vi "Main.vi"() -> ()   [LabVIEW 2013]
doc: "This template is for the Queued Message Handler design pattern.\n\nThe Event Handling Loop generates messages based on user interface actions.\n\nThe Message Handling Loop processes messages generated by the Event Handling Loop, or by other messages. The messages are string values, so new messages can be added easily to the Message Cases case structure in the Message Handling Loop. Each message cluster can also provide an optional value for Message Data, which is a variant that can be converted to whatever message-specific data is required."
uses:
  <vilib>/vision/Image Controls.llb/IMAQ Image.ctl
  Message Passing/MsgQ Loops enum.ctl
  Image Processing/Mask ROI FG Enum.ctl
  System Status/Status FG Enum.ctl
  Globals/Average Sector Data.vi
  controls/UI Data.ctl
  Message Queue/Message Queue.lvlib
  User Event - Stop/User Event - Stop.lvlib
  FPGA/FPGA Frame Grabbing.lvlib
  Image Processing/Image Processing.lvlib
  Common/State Machines/State Machine Lib.lvlib
  Message Passing/Main MsgQ.lvlib
  Common/GUI/GUI.lvlib
  <vilib>/rvi/interface/nirviReadWriteControl/nirviReadWriteControl.xnode
  FGs/FPGA_Reference.ctl
  FPGA Bitfiles/Simulation_WBA.lvbitx
  <vilib>/rvi/errors/niLvFpgaMergeErrorWithErrorCode.vi
  NiFpgaLv.dll
  <vilib>/rvi/errors/niLvFpgaAdjustHostInterfaceError.vi
panel:
  out "Analysis Ticks":u32
  out "Accumulate Ticks":u32
  out "FPGA Display Image":T1(plugin-control)
  out "Right Wingbeat Avg Graph":u8[](graph)
  in  "Start Serial Server":bool=TRUE
  out "Left Wingbeat Avg Graph":u8[](graph)
  in  "Stop Charts":bool
  in  "Wing ROIs":T2
  out "FPGA image info":T5={"Image Type"=0, "Unit"=enum."Undefined", "X Resolution"=2040, "Y Resolution"=1088, "X Step"=1.0, "Y Step"=1.0, "Image Name"="Image"} {"Image Type" items=["Grayscale (U8)", "Grayscale (I16)", "Grayscale (SGL)", "Complex (CSG)", "RGB (U32)", "HSL (U32)", "RGB (U64)", "Grayscale (U16)"]}
  in  "Stream?":bool
  out "FPGA Image":T1
  in  "Test Visual Response":bool
  in  "Test FPGA":bool
  out "Status Update":string="VI Stopped"
  in  "Define Mask":bool
  in  "Acquire Image":bool
  in  "Stop":bool
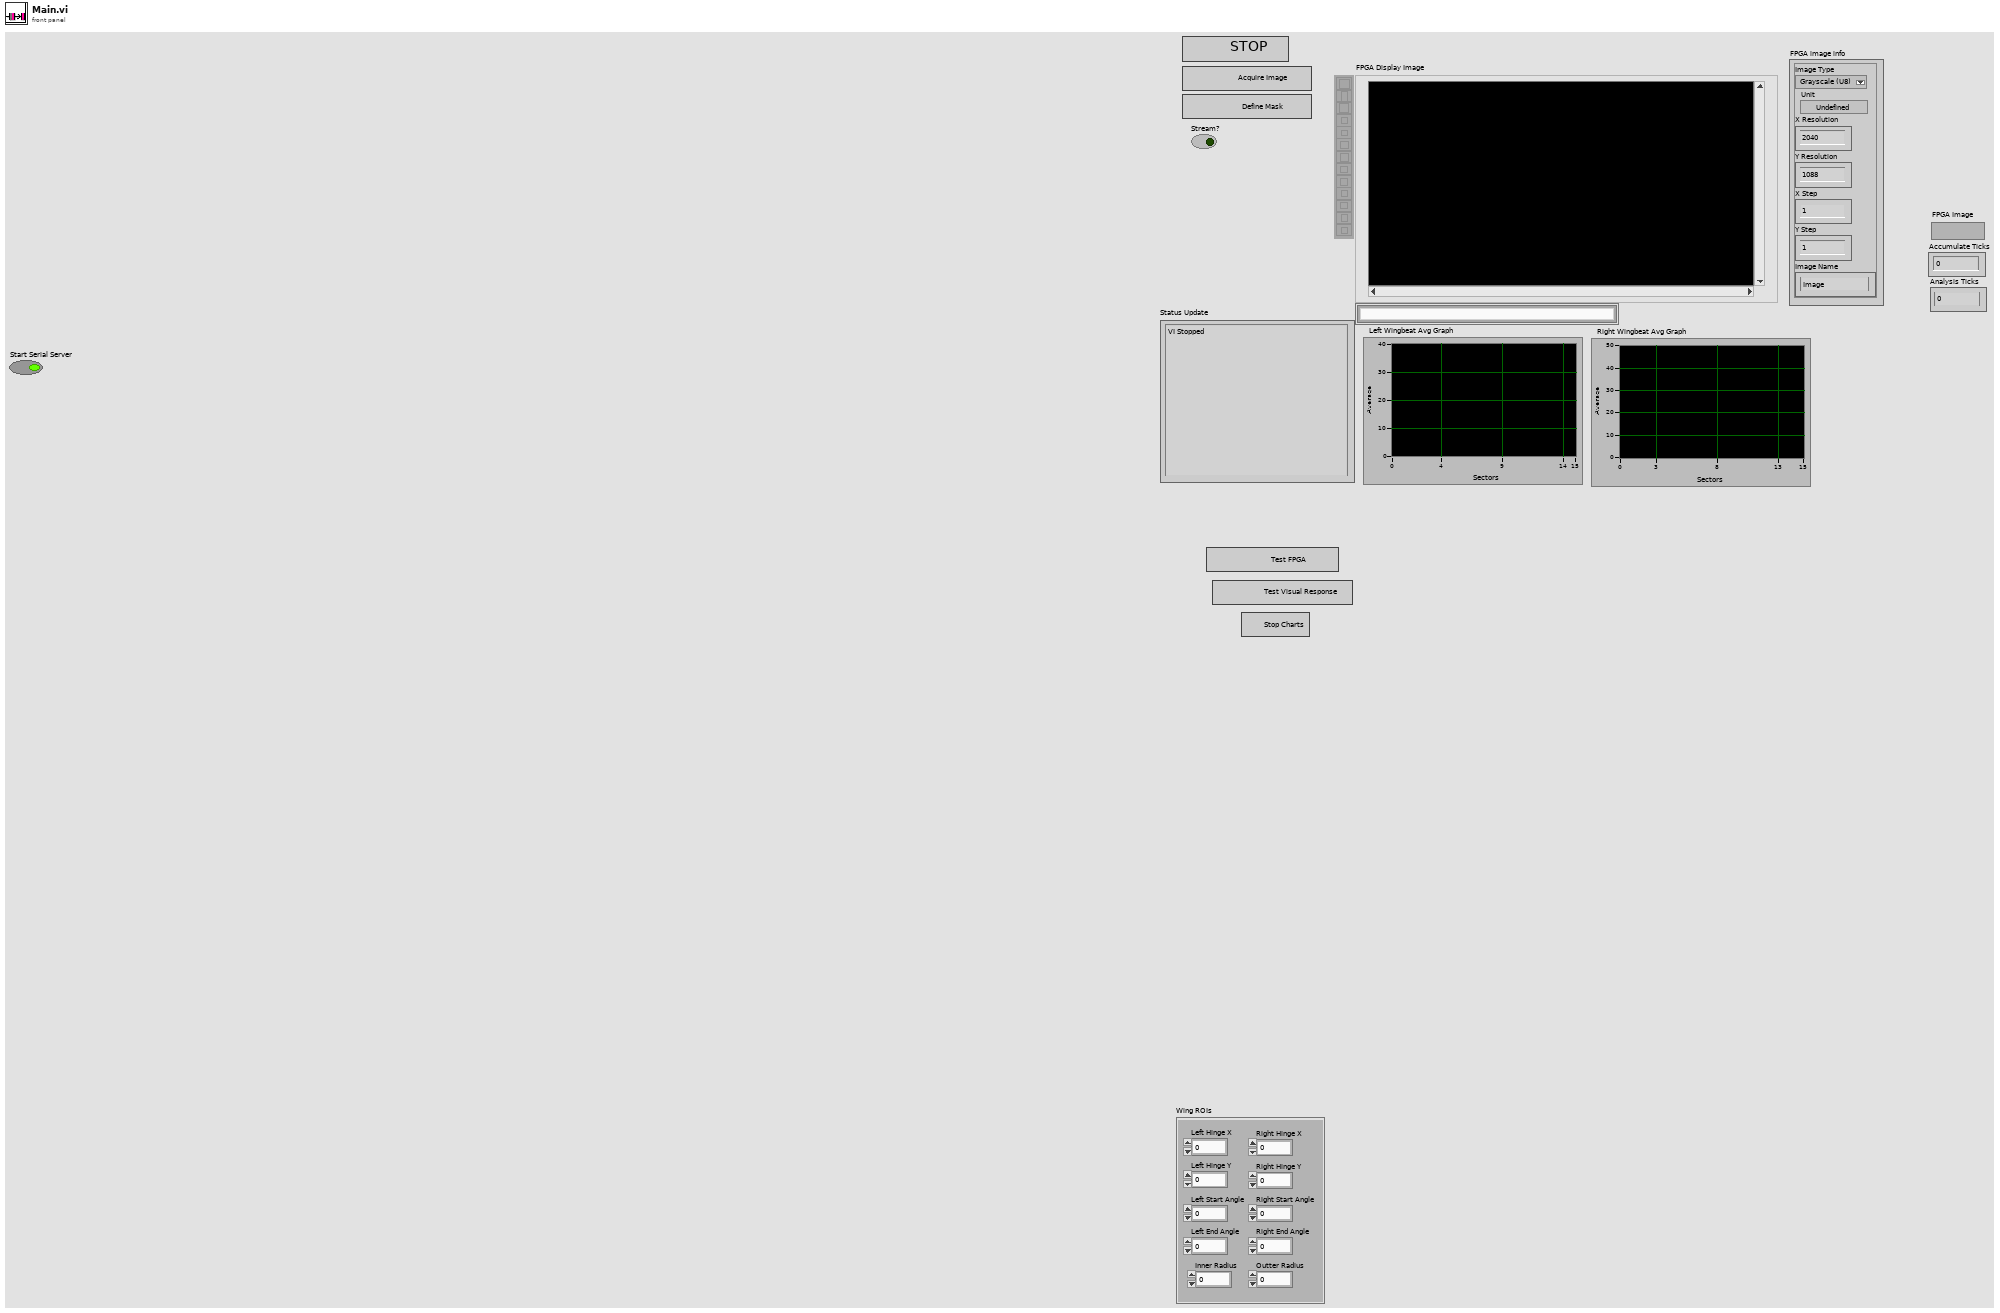
[diagram p1: front panel]
types:
  T1 = typedef "IMAQ Image.ctl" = refnum<image>
  T2 = cluster{"Left Hinge X":u16, "Left Hinge Y":u16, "Inner Radius":u16, "Outter Radius":u16, "Right Hinge X":u16, "Right Hinge Y":u16, "Right Start Angle":i16, "Right End Angle":i16, "Left Start Angle":i16, "Left End Angle":i16}
  T3 = typedef "Image Type" = u32
  T4 = typedef "Image Unit" = enum32{"Undefined", "Angström", "Micrometer", "Millimeter", "Centimeter", "Meter", "Kilometer", "Microinch", "Inch", "Feet", "Nautical miles", "Standard miles", "Steps"}
  T5 = cluster{"Image Type":T3, "Unit":T4, "X Resolution":i32, "Y Resolution":i32, "X Step":sgl, "Y Step":sgl, "Image Name":string}
  T6 = typedef "State Machine Lib.lvlib/STATE cluster.ctl" = cluster{"State":string, "Parameters":variant}
  T7 = typedef "Main MsgQ.lvlib/MsgQ Loops enum.ctl" = enum16{"User Interface", "Image Acq"}
  T8 = typedef "Status FG Enum.ctl" = enum16{"Reset", "Read", "Write"}
  T9 = typedef "Mask ROI FG Enum.ctl" = enum16{"Read", "Write"}
  T10 = typedef "FPGA_Reference.ctl" = refnum<k20>
  T11 = typedef "Mask ROI Cluster.ctl" = cluster{"left annulus":T12, "right annulus":T12, "Threshold Range":cluster{"Lower value":dbl, "Upper value":dbl}, "[Avg BG]":u8[], "Number of Sectors":u8, "Left ROI":T13, "Right ROI":T13, "Left Start Angle Duty Cycle":fxp<+,8,0>, "Left End Angle Duty Cycle":fxp<+,8,0>, "Right End Angle Duty Cycle":fxp<+,8,0>, "Right Start Angle Duty Cycle":fxp<+,8,0>, "[Sector ROIs]":T13[]}
  T12 = typedef "IMAQ Circle" = cluster{"Center X":i32, "Center Y":i32, "Inner Radius":i32, "Outer Radius":i32, "Start Angle":dbl, "End Angle":dbl}
  T13 = typedef "ROI Descriptor" = cluster{"Global Rectangle":i32[], "Contours":cluster{"ID":enum32{"External", "Internal"}, "Type":u32, "Coordinates":i32[]}[]}
  T14 = typedef "UI Data.ctl" = cluster{"Boolean <Replace Me>":bool, "Initial Message":string, "Numeric <Replace Me>":dbl, "Acquire Image Ref":refnum<vi>, "Define Mask Ref":refnum<vi>, "Status Update Ref":refnum<vi>, "Stop Button Ref":refnum<vi>, "FPGA Image":T1, "Processed Image":T1, "Left Annulus":cluster{"Center X":i32, "Center Y":i32, "Inner Radius":i32, "Outer Radius":i32, "Start Angle":dbl, "End Angle":dbl}, "Right Annulus":cluster{"Center X":i32, "Center Y":i32, "Inner Radius":i32, "Outer Radius":i32, "Start Angle":dbl, "End Angle":dbl}}
  T15 = typedef "Message Queue.lvlib/All Message Queues.ctl" = cluster{"UI":refnum<queue>}
  T16 = cluster{"Center X":i32, "Center Y":i32, "Inner Radius":i32, "Outer Radius":i32, "Start Angle":dbl, "End Angle":dbl}
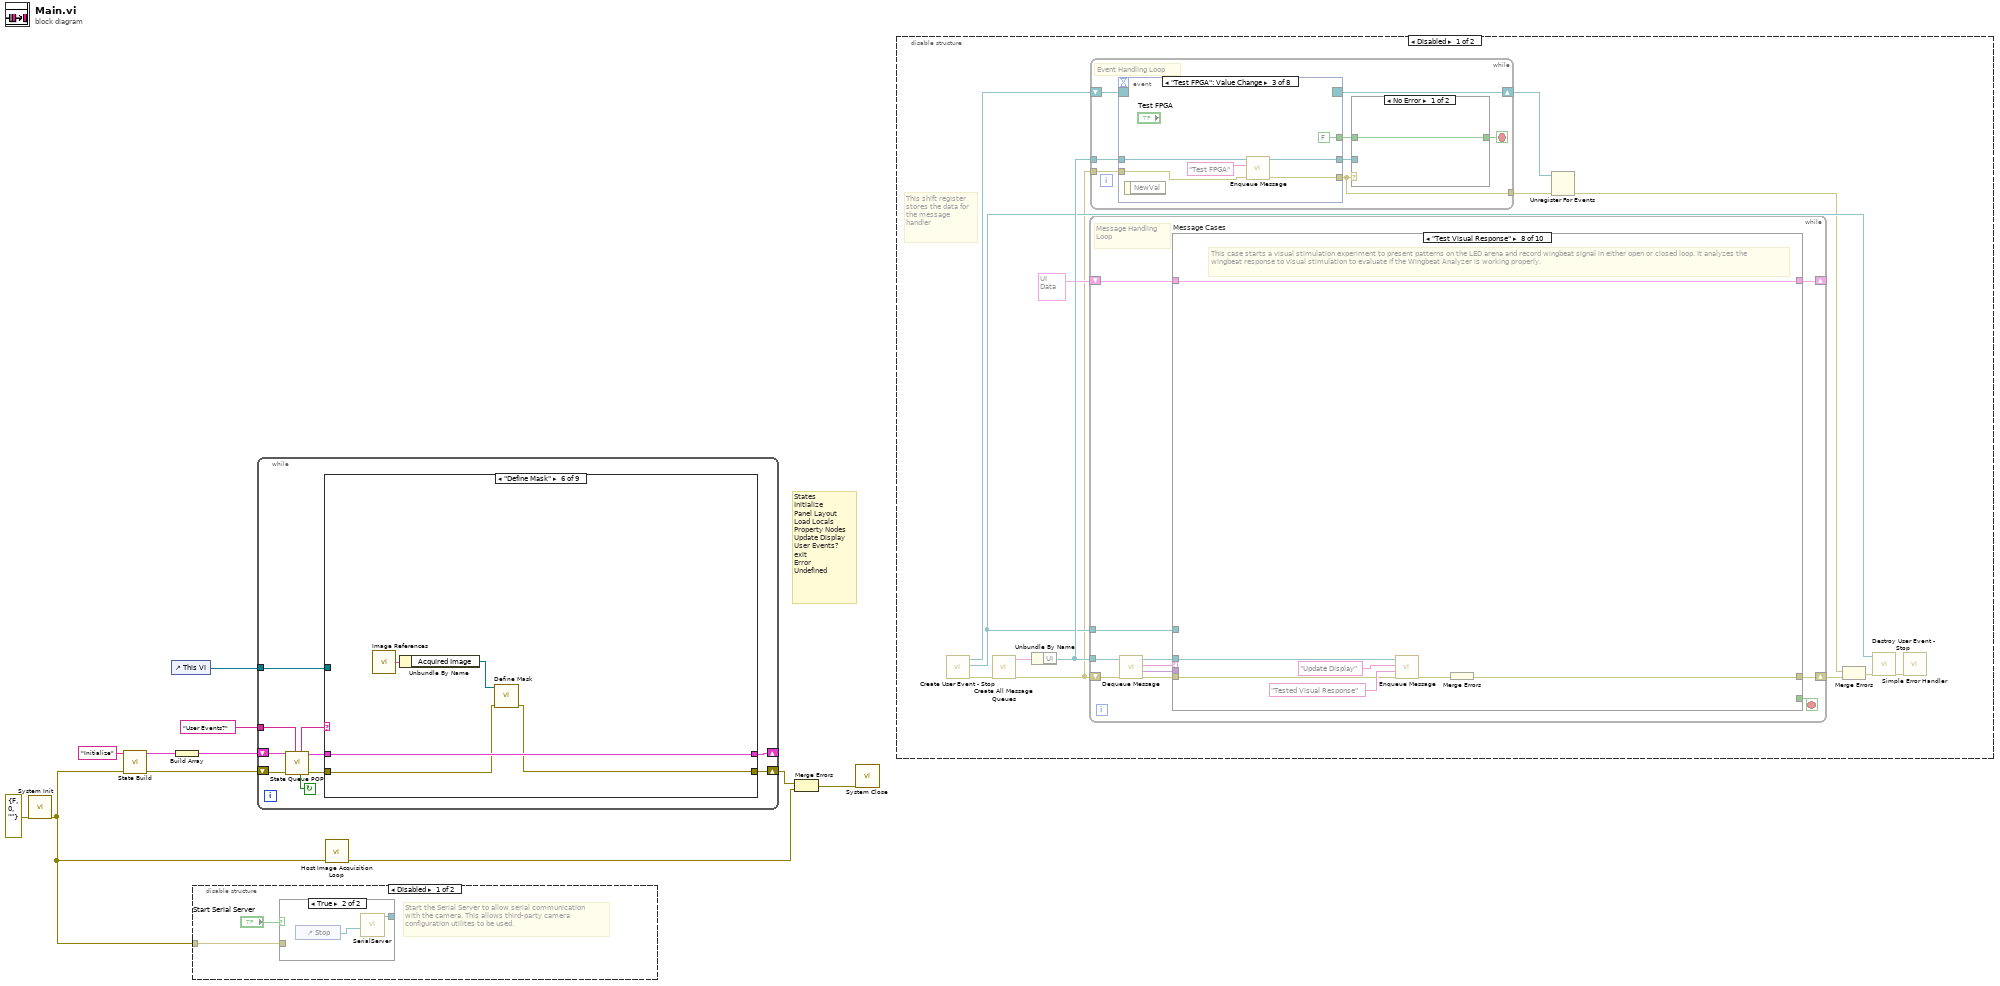
[diagram p0: block diagram]
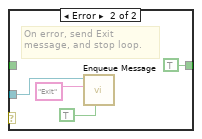
[diagram p4: hidden frame]
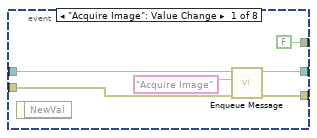
[diagram p5: hidden frame]
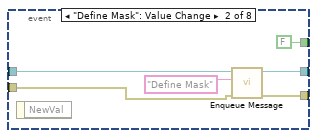
[diagram p6: hidden frame]
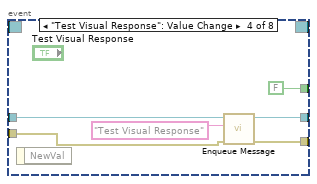
[diagram p7: hidden frame]
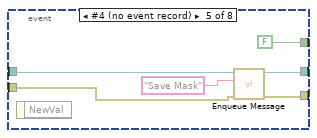
[diagram p8: hidden frame]
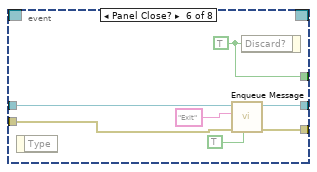
[diagram p9: hidden frame]
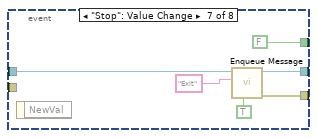
[diagram p10: hidden frame]
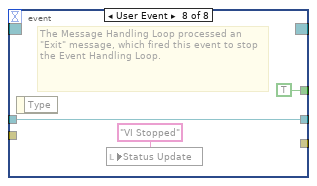
[diagram p11: hidden frame]
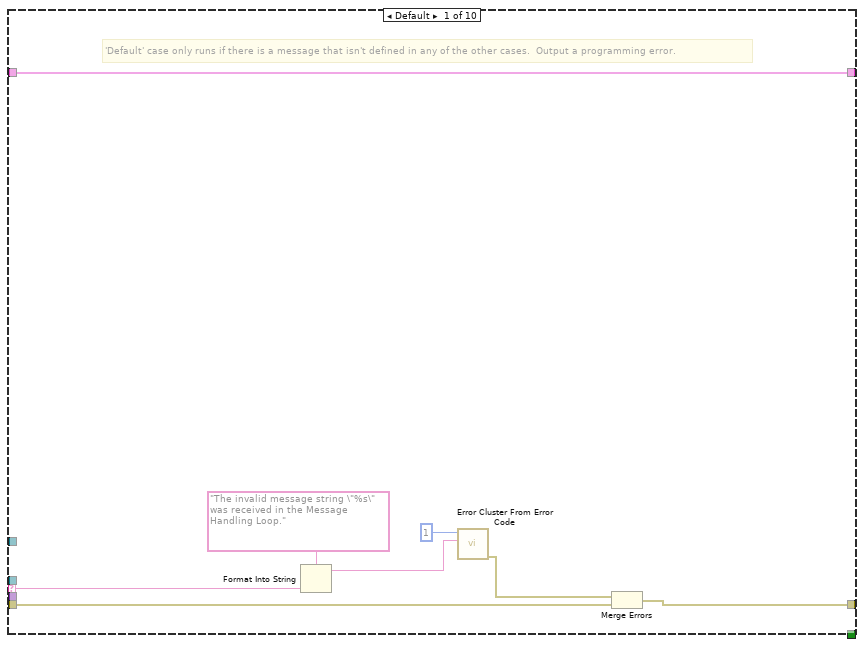
[diagram p12: hidden frame]
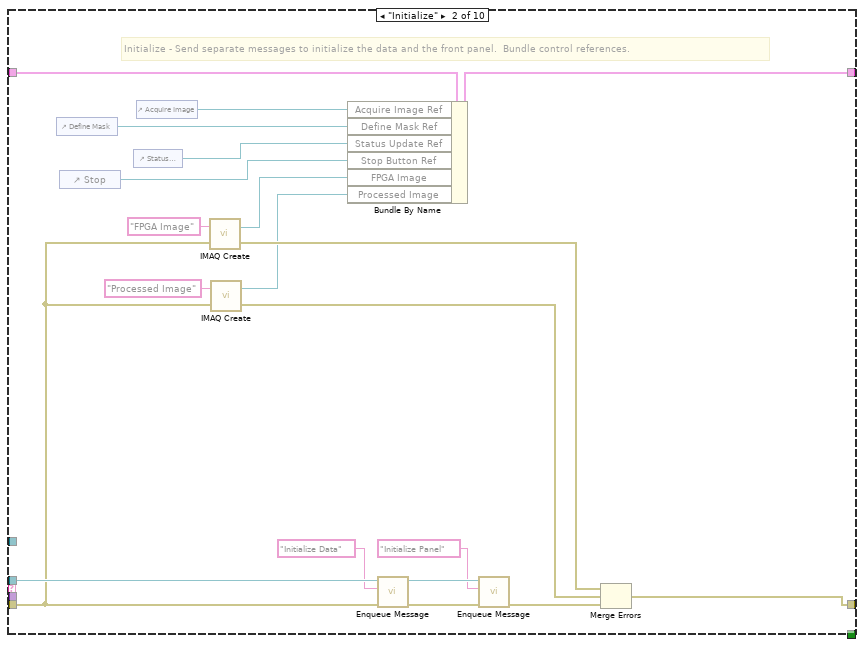
[diagram p13: hidden frame]
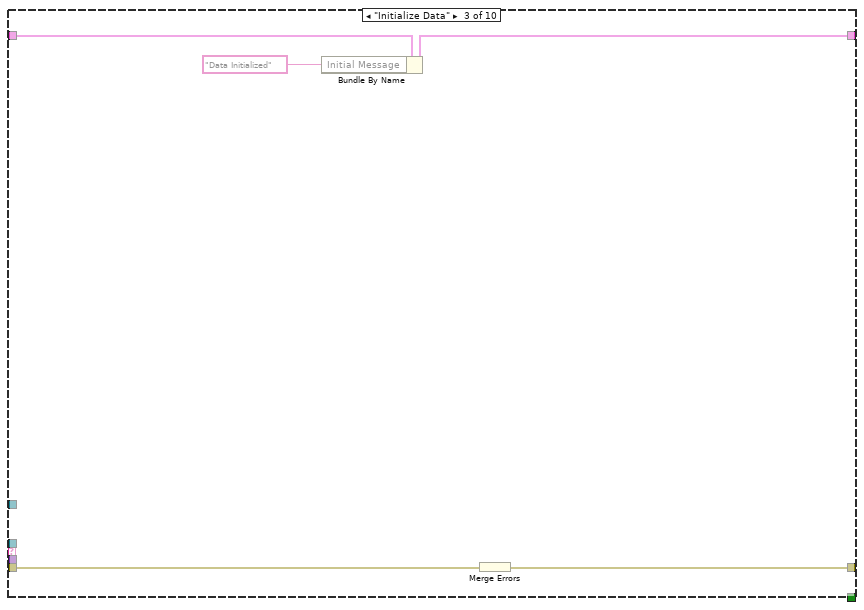
[diagram p14: hidden frame]
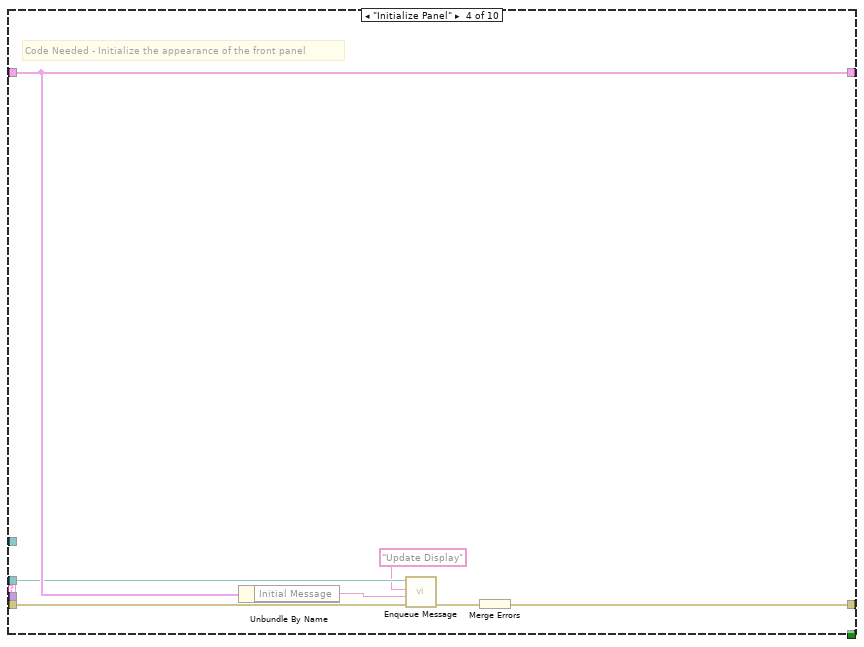
[diagram p15: hidden frame]
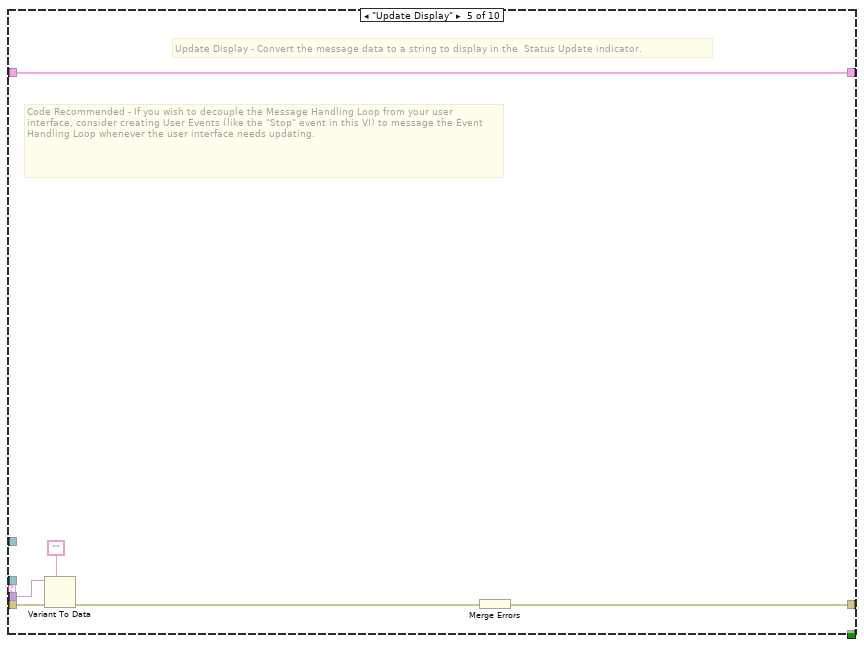
[diagram p16: hidden frame]
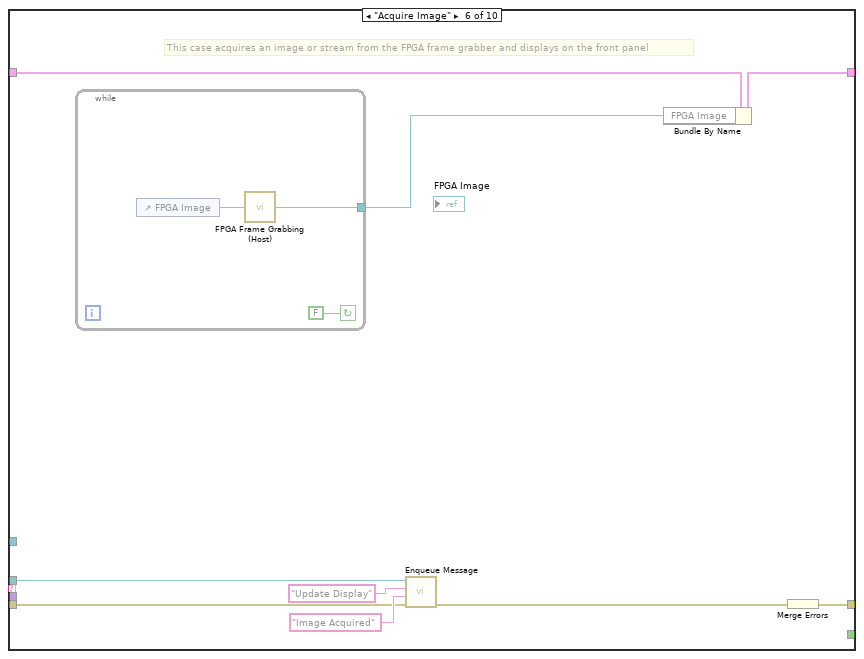
[diagram p17: hidden frame]
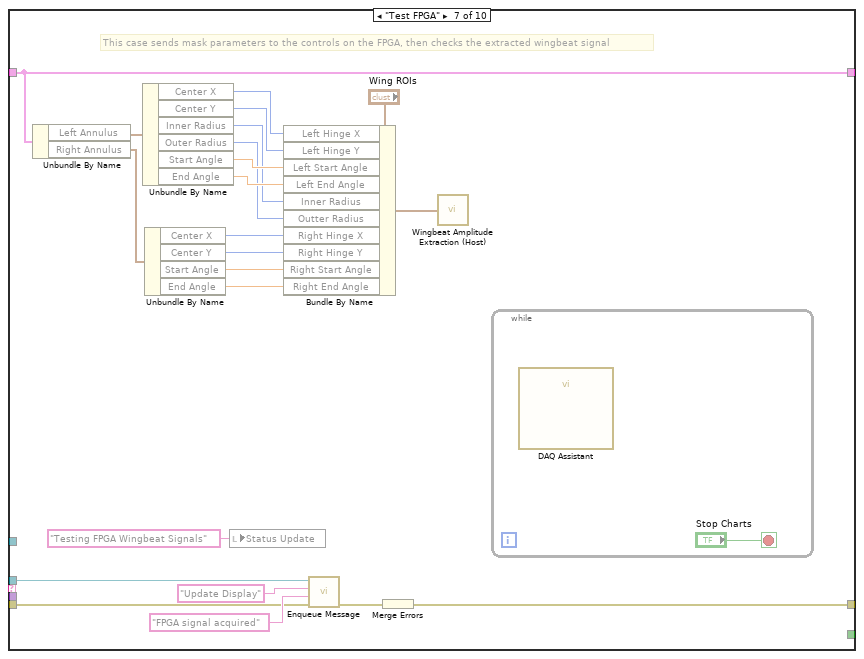
[diagram p18: hidden frame]
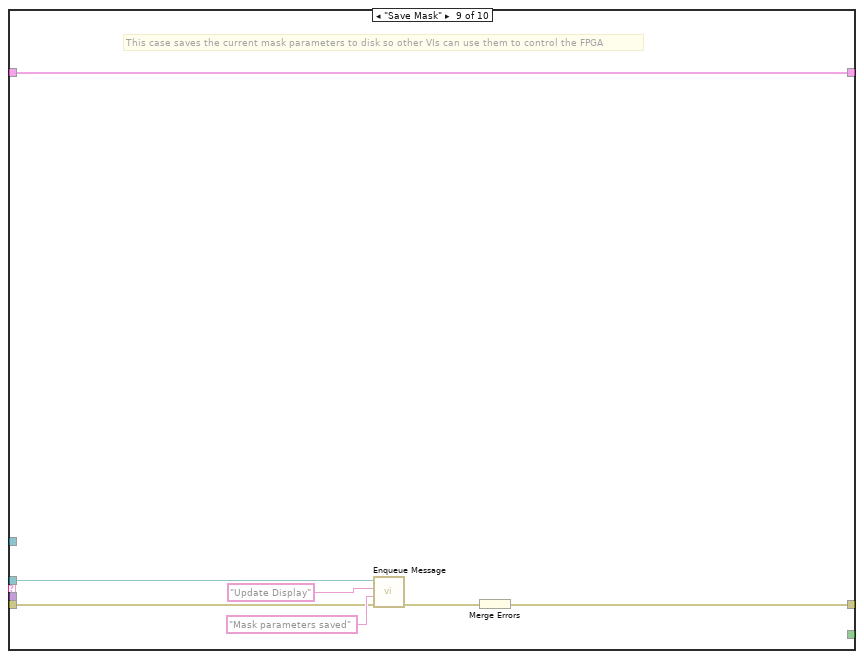
[diagram p19: hidden frame]
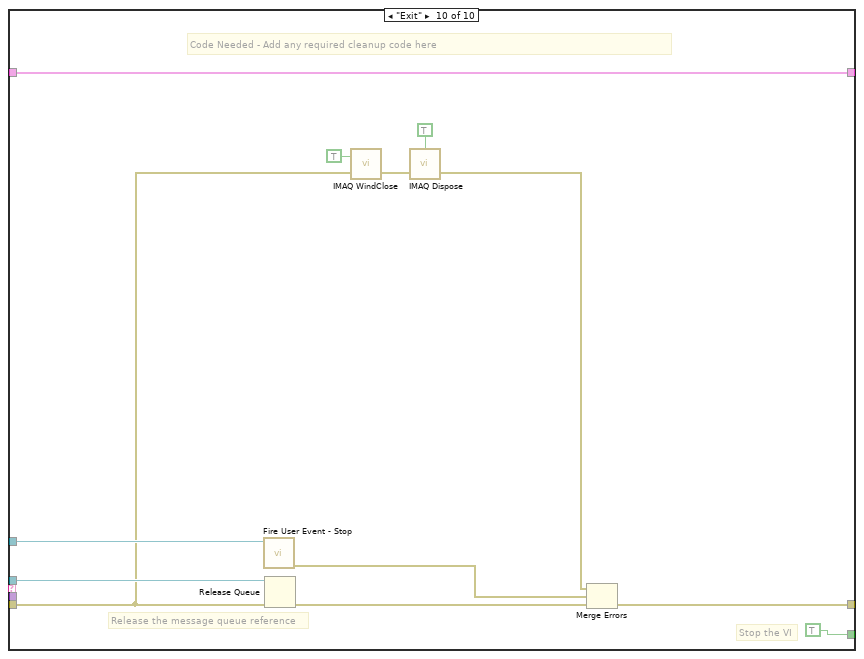
[diagram p20: hidden frame]
diagram:
  # "States\nInitialize\nPanel Layout\nLoad Locals\nProperty Nodes\nUpdate Display\nUser Events?\nexit\nError\nUndefined"
  n1 = call "System Init.vi"("error in (no error)"=errorcluster {"status"=FALSE, "code"=0, "source"=""}) -> ("error out"=w10:errorcluster)  [unwired: 10 in]
  n2 = call "State Build.vi"("error in (no error)"=w10, "State"="Initialize") -> ("error out"=w6:errorcluster, "State Out"=w8:T6)  [unwired: 8 in]
  n3 = control-ref of="This VI"() -> (w4:refnum<vi>)
  n4 = Build Array(w8) -> (w7:T6[])
  n5 = disable-structure shown="Disabled" {
    disable-tunnel: w10 -> [w12 _]
    frame Disabled {
      # "Start the Serial Server to allow serial communication\nwith the camera. This allows third-party camera\nconfiguration utilites to be used."
      n6 = case shown="True" "Start Serial Server" {
        tunnel: [_ w15] -> _
        tunnel: w12 -> [_ _]
        frame False {
        }
        frame True {
          n7 = control-ref of="Stop"() -> (w14:refnum<vi>)
          n8 = call "SerialServer.vi"("Stop Refnum"=w14) -> ("FPGA VI Reference Out"=w15:refnum<k20>)  [unwired: 6 in]
        }
      }
    }
    frame Enabled {
    }
  }
  n9 = while {
    shift-right: [w19] -> _
    shift-left: w7 -> [w25]
    shift-right: [w17] -> w3
    shift-left: w6 -> [w24]
    tunnel: "User Events?" ("State") -> [w22]
    tunnel: w4 -> [w20]
    stop <- w23 continue-if-true
    n10 = call "State Queue POP.vi"("Default state"=w22, "error in (no error)"=w24, "State que in"=w25) -> ("error out"=w16:errorcluster, "State que out"=w18:T6[], "Not Exit?"=w23:bool, "State case out"=w21:string)  [unwired: 4 in, 1 out]
    n11 = case shown="\"Define Mask\"" w21 {
      tunnel: w20 -> [_ _ w36 _ _ _ _ _ _]
      tunnel: [w27 w28 w33 w39 w41 w46 w50 w82 w109] -> w19
      tunnel: w18 -> [w27 w31 w33 w39 w41 w46 w49 _ w109]
      tunnel: [w26 w29 w34 w37 w40 w44 w48 w81 w107] -> w17
      tunnel: w16 -> [w26 w30 w35 w37 w40 w45 w47 w83 w91]
      frame Default {
      }
      frame "Initialize" {
        n12 = call "State Queue PUSH multiple states no parameters.vi"("States to queue"=string[] ["Panel Layout", "Load Locals", "Property Nodes", "Update Display"], "error in (no error)"=w30, "State que in"=w31) -> ("error out"=w29:errorcluster, "State que out"=w28:T6[])  [unwired: 7 in]
      }
      frame "Panel Layout" {
        # "Reset origin to 0,0"
        n13 = call "Reset all pane origins.vi"("error in (no error"=w35, "Vi Ref In"=w36) -> ("error out"=w34:errorcluster)  [unwired: 8 in, 1 out]
      }
      frame "Load Locals" {
        n14 = local write "Stream?"(FALSE ("Stream?")) -> ()
      }
      frame "Property Nodes" {
      }
      frame "Define Mask" {
        n15 = call "Image References.vi"() -> ("Images"=w42:cluster{"Acquired Image":T1, "Display Image":T1})  [unwired: 10 in, 1 out]
        n16 = Unbundle By Name(w42) -> ("Acquired Image"=w43:T1)
        n17 = call "Define Mask.vi"("error in (no error)"=w45, "FPGA Image"=w43) -> ("error out"=w44:errorcluster)  [unwired: 9 in]
      }
      frame "User Events?" {
        n18 = event shown="[3] \"Define Mask\": Value Change" {
          selector: _ -> [_ _ _ _ _]
          dyn-events: _ -> [_ _ _ _ _]
          timeout: 200 -> [_ _ _ _ _]
          tunnel: [w53 w63 w66 w73 w76] -> w50
          tunnel: w49 -> [w54 w63 w66 w75 w79]
          tunnel: [w55 w60 w67 w72 w77] -> w48
          tunnel: w47 -> [w56 w61 w68 w74 w78]
          event Timeout {
            n19 = event-data() -> ()  [unwired: 1 in, 3 out]
            n20 = disable-structure shown="Enabled" {
              frame Disabled {
                n21 = call "FPGA Reference FG.vi"() -> ("FPGA VI Reference Out"=w59:T10)  [unwired: 11 in]
                n22 = xnode "Read/Write Control"("FPGA VI Reference In"=w59) -> ("Accumulate Ticks"=→"Accumulate Ticks", "Analysis Ticks"=→"Analysis Ticks":u32)  [unwired: 1 in, 2 out]
              }
              frame Enabled {
              }
            }
            n23 = call "State Queue PUSH.vi"("State case"="Update Display", "error in (no error)"=w56, "State que in"=w54) -> ("error out"=w55:errorcluster, "State que out"=w53:T6[])  [unwired: 7 in]
          }
          event "Acquire Image": Value Change {
            n24 = event-data() -> ()  [unwired: 1 in, 6 out]
            n25 = call "Send MsgQ.vi"("error in (no error)"=w61, "Message String"="Acquire Single Image", "Send to MsgQ"=MsgQ_Loops_enum."Image Acq") -> ("error out"=w60:errorcluster)  [unwired: 8 in]
          }
          event "Stream?": Value Change {
            n26 = event-data() -> ("NewVal"=w65:bool)  [unwired: 1 in, 5 out]
            n27 = call "Send MsgQ.vi"("error in (no error)"=w68, "Data In"=w65, "Message String"="Stream Image", "Send to MsgQ"=MsgQ_Loops_enum."Image Acq") -> ("error out"=w67:errorcluster)  [unwired: 7 in]
          }
          event "Define Mask": Value Change {
            n28 = event-data() -> ()  [unwired: 1 in, 6 out]
            n29 = call "State Queue PUSH.vi"("State case"="Define Mask", "error in (no error)"=w74, "State que in"=w75) -> ("error out"=w72:errorcluster, "State que out"=w73:T6[])  [unwired: 7 in]
          }
          event "Stop": Value Change {
            n30 = event-data() -> ()  [unwired: 1 in, 6 out]
            n31 = call "State Queue PUSH.vi"("State case"="exit", "error in (no error)"=w78, "State que in"=w79) -> ("error out"=w77:errorcluster, "State que out"=w76:T6[])  [unwired: 7 in]
          }
        }
      }
      frame "exit" {
        n32 = call "Broadcast Exit.vi"("error in"=w83) -> ("error out"=w81:errorcluster)  [unwired: 10 in]
        n33 = call "Queue EXIT state.vi"() -> ("Exit State Q"=w82:T6[])  [unwired: 1 in]
      }
      frame "Update Display" {
        n34 = call "Image References.vi"() -> ("Images"=w87:cluster{"Acquired Image":T1, "Display Image":T1})  [unwired: 10 in, 1 out]
        n35 = call "Status FG.vi"("Operation"=Status_FG_Enum."Read") -> ("Status Out"=→"Status Update":string)  [unwired: 9 in, 1 out]
        n36 = call "Mask ROI FG.vi"("Operation"=Mask_ROI_FG_Enum."Read") -> ("Mask ROI Out"=w104:T11)  [unwired: 9 in, 1 out]
        n37 = Unbundle By Name(w87) -> ("Acquired Image"=w86:T1, "Display Image"=w85:T1)
        n38 = Unbundle By Name(w104) -> ("Number of Sectors"=w101:u8)
        n39 = global read "Average Sector Data.vi" "[Average Sector Data]"() -> (w106:u8[])
        n40 = call "Overlay Image with Sector ROI.vi"("FPGA Display Image In"=w85, "error in"=w91, "FPGA Image"=w86) -> ("error out"=w90:errorcluster, "FPGA Display Image Out"=→"FPGA Display Image":T1)  [unwired: 7 in]
        n41 = call "IMAQ GetImageInfo"("error in (no error)"=w90, "Image"=w86) -> ("error out"=w108:errorcluster, "X Step"=w96:sgl, "Y Resolution"=w95:i32, "X Resolution"=w94:i32, "Y Step"=w97:sgl, "Unit"=w93:T4, "Image Name"=w98:string, "Image Type"=w92:T3)  [unwired: 2 in]
        n42 = Split 1D Array(array=w106, index=w101) -> (first subarray=→"Left Wingbeat Avg Graph":u8[], second subarray=→"Right Wingbeat Avg Graph":u8[])
        n43 = local read "FPGA image info"() -> (w100:T5)
        n44 = Bundle By Name(cluster=w100, "Image Type"=w92, "Unit"=w93, "X Resolution"=w94, "Y Resolution"=w95, "X Step"=w96, "Y Step"=w97, "Image Name"=w98) -> (→"FPGA image info":T5)
        n45 = call <vilib>:"Clear Errors.vi"("error in (no error)"=w108) -> ("error out"=w107:errorcluster)  [unwired: 6 in]
      }
    }
  }
  n46 = call "Host Image Acquisition Loop.vi"("error in"=w10) -> ("error out"=w2:errorcluster)  [unwired: 10 in]
  n47 = Merge Errors(w3, w2) -> (w1:errorcluster)
  n48 = call "System Close.vi"("error in (no error)"=w1) -> ()  [unwired: 10 in, 1 out]
  n49 = disable-structure shown="Disabled" {
    frame Disabled {
      # "This shift register\nstores the data for the message handler"
      n50 = call "Create User Event - Stop.vi"() -> ("error out"=w118:errorcluster, "User Event - Stop"=w115:refnum<user-event>, "Stop Event Registration Refnum"=w119:refnum<event-registration>)  [unwired: 9 in]
      n51 = call "Create All Message Queues.vi"("error in (no error)"=w118) -> ("error out"=w110:errorcluster, "Message Queues out"=w122:T15)  [unwired: 9 in]
      n52 = Unbundle By Name(w122) -> ("UI"=w120:refnum<queue>)
      n53 = while {
        tunnel: w120 -> [w182]
        shift-right: [w191] -> _
        shift-left: T14 {"Boolean <Replace Me>"=TRUE, "Initial Message"="", "Numeric <Replace Me>"=0.0, "Acquire Image Ref"=refnum, "Define Mask Ref"=refnum, "Status Update Ref"=refnum, "Stop Button Ref"=refnum, "FPGA Image"=refnum, "Processed Image"=refnum, "Left Annulus"={"Center X"=0, "Center Y"=0, "Inner Radius"=0, "Outer Radius"=0, "Start Angle"=0.0, "End Angle"=0.0}, "Right Annulus"={"Center X"=0, "Center Y"=0, "Inner Radius"=0, "Outer Radius"=0, "Start Angle"=0.0, "End Angle"=0.0}} ("Data Cluster") -> [w192]
        tunnel: w115 -> [w188]
        shift-right: [w189] -> w121
        shift-left: w110 -> [w187]
        stop <- w190 stop-if-true
        # "Message Handling Loop"
        n54 = call "Dequeue Message.vi"("error in (no error)"=w187, "Message Queue"=w182) -> ("error out"=w186:errorcluster, "Message Data"=w184:variant, "Message"=w185:string, "dup Message Queue"=w183:refnum<queue>)  [unwired: 6 in]
        n55 = case "Message Cases" shown="\"Test Visual Response\"" w185 {
          selector: w185 -> [w198 _ _ _ _ _ _ _ _ _]
          tunnel: w183 -> [_ w218 _ w229 _ w246 w269 w277 w285 w301]
          tunnel: w186 -> [w195 w203 w225 w230 w237 w241 w270 w278 w283 w290]
          tunnel: [w193 w205 w221 w231 w238 w248 w268 w276 w288 w297] -> w189
          tunnel: w192 -> [w200 w215 w224 w232 w239 w243 w267 w282 w289 w300]
          tunnel: [w200 w214 w223 w232 w239 w242 w267 w282 w289 w300] -> w191
          tunnel: [_ _ _ _ _ _ _ _ _ TRUE] -> w190
          tunnel: w184 -> [_ _ _ _ w236 _ _ _ _ _]
          tunnel: w188 -> [_ _ _ _ _ _ _ _ _ w296]
          frame Default {
            # "'Default' case only runs if there is a message that isn't defined in any of the other cases.  Output a programming error."
            n56 = Format Into String(format string="The invalid message string \"%s\" was received in the Message Handling Loop." ("Unknown Message Error Text"), w198) -> (resulting string=w196:string)  [unwired: 2 in, 1 out]
            n57 = call <vilib>:"Error Cluster From Error Code.vi"("error message (\"\")"=w196, "error code (0)"=1) -> ("error out"=w194:errorcluster)  [unwired: 7 in]
            n58 = Merge Errors(w194, w195) -> (w193:errorcluster)
          }
          frame "Initialize" {
            # "Initialize - Send separate messages to initialize the data and the front panel.  Bundle control references."
            n59 = control-ref of="Define Mask"() -> (w212:refnum<vi>)
            n60 = control-ref of="Stop"() -> (w210:refnum<vi>)
            n61 = control-ref of="Status Update"() -> (w211:refnum<vi>)
            n62 = control-ref of="Acquire Image"() -> (w213:refnum<vi>)
            n63 = call "IMAQ Create"("Image Name"="FPGA Image", "error in (no error)"=w203) -> ("New Image"=w208:T1, "error out"=w204:errorcluster)  [unwired: 3 in]
            n64 = call "IMAQ Create"("Image Name"="Processed Image", "error in (no error)"=w203) -> ("New Image"=w201:T1, "error out"=w202:errorcluster)  [unwired: 3 in]
            n65 = Bundle By Name(cluster=w215, "Acquire Image Ref"=w213, "Define Mask Ref"=w212, "Status Update Ref"=w211, "Stop Button Ref"=w210, "FPGA Image"=w208, "Processed Image"=w201) -> (w214:T14)
            n66 = call "Enqueue Message.vi"("error in (no error)"=w203, "Message"="Initialize Data", "Message Queue"=w218) -> ("error out"=w220:errorcluster, "dup Message Queue"=w219:refnum<queue>)  [unwired: 7 in]
            n67 = call "Enqueue Message.vi"("error in (no error)"=w220, "Message"="Initialize Panel", "Message Queue"=w219) -> ("error out"=w206:errorcluster)  [unwired: 7 in, 1 out]
            n68 = Merge Errors(w204, w202, w206) -> (w205:errorcluster)
          }
          frame "Initialize Data" {
            n69 = Bundle By Name(cluster=w224, "Initial Message"="Data Initialized") -> (w223:T14)
            n70 = Merge Errors(w225) -> (w221:errorcluster)
          }
          frame "Initialize Panel" {
            # "Code Needed - Initialize the appearance of the front panel"
            n71 = Unbundle By Name(w232) -> ("Initial Message"=w226:string)
            n72 = call "Enqueue Message.vi"("error in (no error)"=w230, "Message Data"=w226, "Message"="Update Display", "Message Queue"=w229) -> ("error out"=w228:errorcluster)  [unwired: 6 in, 1 out]
            n73 = Merge Errors(w228) -> (w231:errorcluster)
          }
          frame "Update Display" {
            # "Code Recommended - If you wish to decouple the Message Handling Loop from your user interface, consider creating User Events (like the \"Stop\" event in this VI) to message the Event Handling Loop whenever the user interface needs updating."
            # "Update Display - Convert the message data to a string to display in the  Status Update indicator."
            n74 = Variant To Data(error in=w237, type="", Variant=w236) -> (data=w233:string, error out=w234:errorcluster)
            n75 = Merge Errors(w234) -> (w238:errorcluster)
          }
          frame "Acquire Image" {
            # "This case acquires an image or stream from the FPGA frame grabber and displays on the front panel"
            n76 = while {
              tunnel: [w251] -> w240
              stop <- FALSE continue-if-true
              n77 = control-ref of="FPGA Image"() -> (w250:refnum<vi>)
              n78 = call "FPGA Frame Grabbing (Host).vi"("Ctl Refnum"=w250) -> ("Image"=w251:T1)
            }
            n79 = call "Enqueue Message.vi"("error in (no error)"=w241, "Message Data"="Image Acquired" ("\"Do Something\" button pressed"), "Message"="Update Display", "Message Queue"=w246) -> ("error out"=w247:errorcluster)  [unwired: 6 in, 1 out]
            n80 = Bundle By Name(cluster=w243, "FPGA Image"=w240) -> (w242:T14)
            n81 = Merge Errors(w247) -> (w248:errorcluster)
          }
          frame "Test FPGA" {
            # "This case sends mask parameters to the controls on the FPGA, then checks the extracted wingbeat signal"
            n82 = Unbundle By Name(w267) -> ("Left Annulus"=w266:T16, "Right Annulus"=w265:T16)
            n83 = Unbundle By Name(w266) -> ("Center X"=w263:i32, "Center Y"=w262:i32, "Inner Radius"=w259:i32, "Outer Radius"=w258:i32, "Start Angle"=w261:dbl, "End Angle"=w260:dbl)
            n84 = Unbundle By Name(w265) -> ("Center X"=w257:i32, "Center Y"=w256:i32, "Start Angle"=w255:dbl, "End Angle"=w254:dbl)
            n85 = local write "Status Update"("Testing FPGA Wingbeat Signals" ("Status Update")) -> ()
            n86 = Bundle By Name(cluster="Wing ROIs", "Left Hinge X"=w263, "Left Hinge Y"=w262, "Left Start Angle"=w261, "Left End Angle"=w260, "Inner Radius"=w259, "Outter Radius"=w258, "Right Hinge X"=w257, "Right Hinge Y"=w256, "Right Start Angle"=w255, "Right End Angle"=w254) -> (w253:T2)
            n87 = call "Enqueue Message.vi"("error in (no error)"=w270, "Message Data"="FPGA signal acquired" ("\"Do Something\" button pressed"), "Message"="Update Display", "Message Queue"=w269) -> ("error out"=w273:errorcluster)  [unwired: 6 in, 1 out]
            n88 = Merge Errors(w273) -> (w268:errorcluster)
            n89 = call "Wingbeat Amplitude Extraction (Host).vi"("Wing ROIs"=w253) -> ()  [unwired: 1 in]
            n90 = while {
              stop <- "Stop Charts" stop-if-true
              n91 = call "DAQ Assistant"() -> ("data"=w274:dynamicdata)  [unwired: 17 in, 2 out]
            }
          }
          frame "Test Visual Response" {
            # "This case starts a visual stimulation experiment to present patterns on the LED arena and record wingbeat signal in either open or closed loop. It analyzes the wingbeat response to visual stimulation to evaluate if the Wingbeat Analyzer is working properly."
            n92 = call "Enqueue Message.vi"("error in (no error)"=w278, "Message Data"="Tested Visual Response" ("\"Do Something\" button pressed"), "Message"="Update Display", "Message Queue"=w277) -> ("error out"=w281:errorcluster)  [unwired: 6 in, 1 out]
            n93 = Merge Errors(w281) -> (w276:errorcluster)
          }
          frame "Save Mask" {
            # "This case saves the current mask parameters to disk so other VIs can use them to control the FPGA"
            n94 = call "Enqueue Message.vi"("error in (no error)"=w283, "Message Data"="Mask parameters saved" ("\"Do Something Else\" button pressed"), "Message"="Update Display", "Message Queue"=w285) -> ("error out"=w284:errorcluster)  [unwired: 6 in, 1 out]
            n95 = Merge Errors(w284) -> (w288:errorcluster)
          }
          frame "Exit" {
            # "Stop the VI"
            # "Release the message queue reference"
            # "Code Needed - Add any required cleanup code here"
            n96 = call "Fire User Event - Stop.vi"("User Event - Stop"=w296) -> ("error out"=w295:errorcluster)  [unwired: 10 in]
            n97 = Release Queue(queue=w301, error in (no error)=w290) -> (error out=w298:errorcluster)  [unwired: 1 in, 2 out]
            n98 = call "IMAQ WindClose"("Close All Windows (False)"=TRUE, "error in (no error)"=w290) -> ("error out"=w292:errorcluster)  [unwired: 4 in]
            n99 = call "IMAQ Dispose"("All Images? (No)"=TRUE, "error in (no error)"=w292) -> ("error out"=w291:errorcluster)  [unwired: 4 in]
            n100 = Merge Errors(w291, w295, w298) -> (w297:errorcluster)
          }
        }
      }
      n101 = while {
        tunnel: w120 -> [w130]
        tunnel: [w126] -> w113
        shift-right: [w124] -> w112
        shift-left: w119 -> [w125]
        tunnel: w110 -> [w123]
        stop <- w128 stop-if-true
        # "Event Handling Loop"
        n102 = event shown="[2] \"Test FPGA\": Value Change" {
          selector: w125 -> [_ _ _ _ _ _ _ _]
          dyn-events: [_ _ _ _ _ _ _ _] -> w124
          timeout: _ -> [_ _ _ _ _ _ _ _]
          tunnel: [FALSE ("Discard?") FALSE ("Discard?") FALSE ("Discard?") FALSE ("Discard?") FALSE ("Discard?") w172 FALSE ("Discard?") TRUE ("Discard?")] -> w129
          tunnel: w130 -> [w141 w147 w153 w158 w163 w171 w178 w181]
          tunnel: [w140 w145 w150 w155 w160 w170 w177 _] -> w126
          tunnel: [w139 w146 w149 w157 w162 w169 w175 w181] -> w127
          tunnel: w123 -> [w137 w143 w151 w154 w161 w166 _ _]
          event "Acquire Image": Value Change {
            n103 = event-data() -> ()  [unwired: 1 in, 1 out]
            n104 = call "Enqueue Message.vi"("error in (no error)"=w137, "Message"="Acquire Image", "Message Queue"=w141) -> ("error out"=w140:errorcluster, "dup Message Queue"=w139:refnum<queue>)  [unwired: 7 in]
          }
          event "Define Mask": Value Change {
            n105 = event-data() -> ()  [unwired: 1 in, 1 out]
            n106 = call "Enqueue Message.vi"("error in (no error)"=w143, "Message"="Define Mask", "Message Queue"=w147) -> ("error out"=w145:errorcluster, "dup Message Queue"=w146:refnum<queue>)  [unwired: 7 in]
          }
          event "Test FPGA": Value Change {
            n107 = event-data() -> ()  [unwired: 1 in, 1 out]
            n108 = call "Enqueue Message.vi"("error in (no error)"=w151, "Message"="Test FPGA", "Message Queue"=w153) -> ("error out"=w150:errorcluster, "dup Message Queue"=w149:refnum<queue>)  [unwired: 7 in]
          }
          event "Test Visual Response": Value Change {
            n109 = event-data() -> ()  [unwired: 1 in, 1 out]
            n110 = call "Enqueue Message.vi"("error in (no error)"=w154, "Message"="Test Visual Response", "Message Queue"=w158) -> ("error out"=w155:errorcluster, "dup Message Queue"=w157:refnum<queue>)  [unwired: 7 in]
          }
          event #4 (no event record) {
            n111 = event-data() -> ()  [unwired: 1 in, 1 out]
            n112 = call "Enqueue Message.vi"("error in (no error)"=w161, "Message"="Save Mask", "Message Queue"=w163) -> ("error out"=w160:errorcluster, "dup Message Queue"=w162:refnum<queue>)  [unwired: 7 in]
          }
          event Panel Close? {
            w172 = TRUE ("Discard?")
            n113 = event-data() -> ()  [unwired: 1 in, 1 out]
            n114 = call "Enqueue Message.vi"("Priority Message? (F)"=TRUE, "error in (no error)"=w166, "Message"="Exit", "Message Queue"=w171) -> ("error out"=w170:errorcluster, "dup Message Queue"=w169:refnum<queue>)  [unwired: 6 in]
            n115 = event-data("Discard?"=w172) -> ()  [unwired: 1 in, 1 out]
          }
          event "Stop": Value Change {
            n116 = event-data() -> ()  [unwired: 1 in, 1 out]
            n117 = call "Enqueue Message.vi"("Priority Message? (F)"=TRUE, "Message"="Exit", "Message Queue"=w178) -> ("error out"=w177:errorcluster, "dup Message Queue"=w175:refnum<queue>)  [unwired: 7 in]
          }
          event User Event {
            # "The Message Handling Loop processed an \"Exit\" message, which fired this event to stop the Event Handling Loop."
            n118 = event-data() -> ()  [unwired: 1 in, 1 out]
            n119 = local write "Status Update"("VI Stopped" ("VI Stopped")) -> ()
          }
        }
        n120 = case shown="No Error" w126 {
          tunnel: [w131 TRUE ("Discard?")] -> w128
          tunnel: w129 -> [w131 _]
          tunnel: w127 -> [_ w134]
          frame No Error {
          }
          frame Error {
            # "On error, send Exit message, and stop loop."
            n121 = call "Enqueue Message.vi"("Priority Message? (F)"=TRUE, "Message"="Exit", "Message Queue"=w134) -> ()  [unwired: 7 in, 2 out]
          }
        }
      }
      n122 = Unregister For Events(event registration refnum=w112, error in=w113) -> (error out=w114:errorcluster)
      n123 = Merge Errors(w114, w121) -> (w116:errorcluster)
      n124 = call "Destroy User Event - Stop.vi"("error in (no error)"=w116, "User Event - Stop"=w115) -> ("error out"=w117:errorcluster)  [unwired: 9 in]
      n125 = call <vilib>:"Simple Error Handler.vi"("error in (no error)"=w117) -> ()  [unwired: 4 in, 5 out]
    }
    frame Enabled {
    }
  }
